vi "vision black line.vi"() -> ()   [LabVIEW 2011]
panel:
  out "Image Out 4":T1(plugin-control)
  in  "Stop (F)":bool
  out "Image Out 2":T1(plugin-control)
  out "Image Out 3":T1(plugin-control)
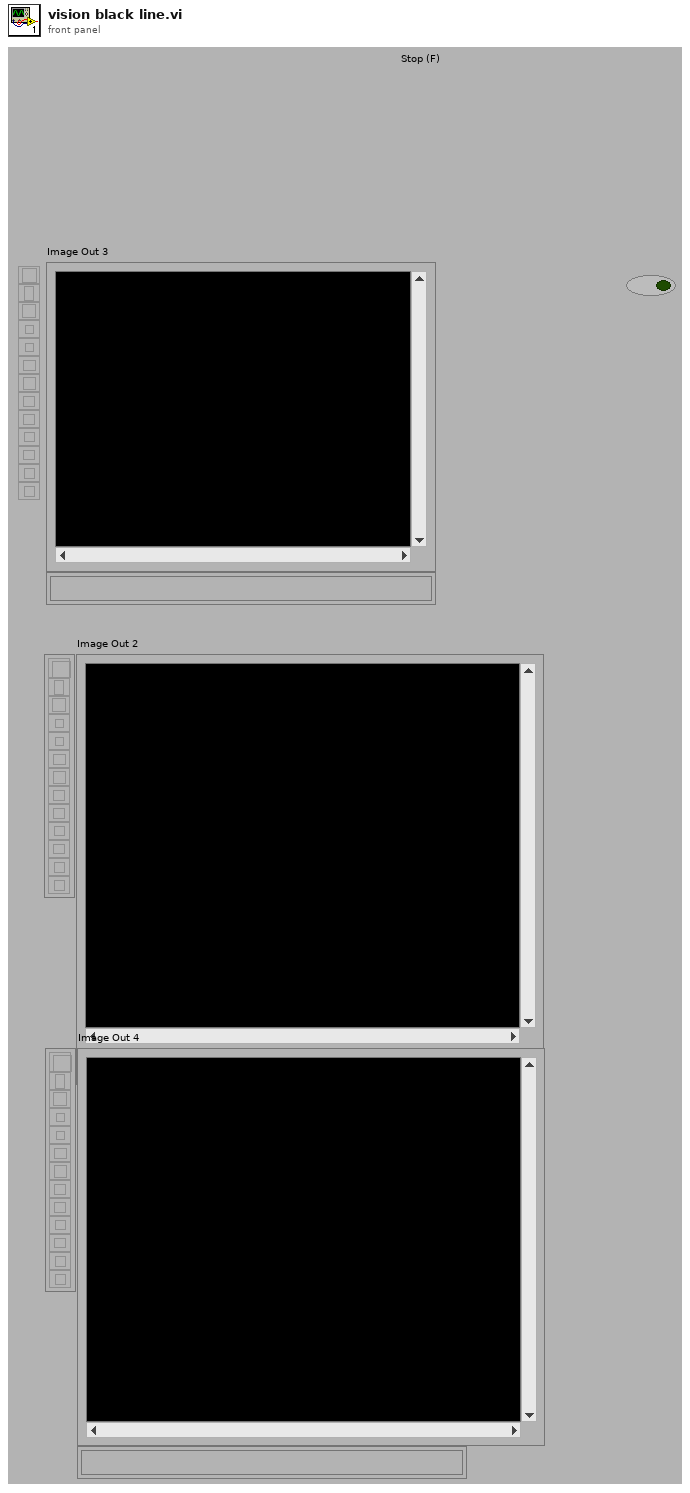
[diagram p1: front panel]
types:
  T1 = typedef "IMAQ Image.ctl" = refnum<image>
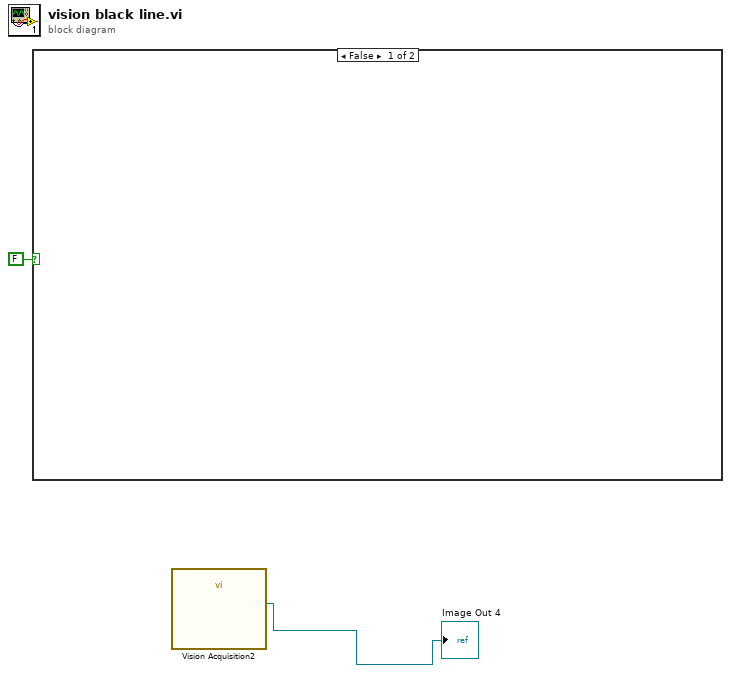
[diagram p0: block diagram]
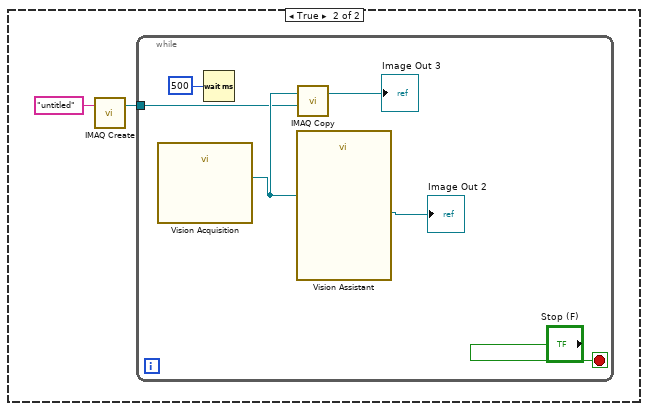
[diagram p2: hidden frame]
diagram:
  n1 = case shown="False" FALSE {
    frame False {
    }
    frame True {
      n2 = call "IMAQ Create"("Image Name"="untitled") -> ("New Image"=w3:T1)  [unwired: 4 in, 1 out]
      n3 = while {
        tunnel: w3 -> [w6]
        stop <- "Stop (F)" stop-if-true
        n4 = call "Vision Acquisition"() -> ("Image Out"=w7:T1)  [unwired: 25 in, 2 out]
        n5 = Wait (ms)(milliseconds to wait=u32 500) -> ()  [unwired: 1 out]
        n6 = call "Vision Assistant"("Image In"=w7) -> ("Image Out"=→"Image Out 2":T1)  [unwired: 25 in, 1 out]
        n7 = call "IMAQ Copy"("Image Dst"=w6, "Image Src"=w7) -> ("Image Dst Out"=→"Image Out 3":T1)  [unwired: 4 in, 1 out]
      }
    }
  }
  n8 = call "Vision Acquisition2"() -> ("Image Out"=→"Image Out 4":T1)  [unwired: 25 in, 2 out]
